vi "D-Lockin_JKISM.vi"(8 "error in (no error)":errorcluster, 11 "SweepControl":refnum<class "SweepControl.lvclass">) -> (0 "error out":errorcluster)   [LabVIEW 2016, in "Transport.lvclass"]
uses:
  Transport.lvclass
  <userlib>/LevyLab/LV to ITX/LVtoITX.lvclass
  SweepControl/SweepControl.lvclass
  Control Experiment/Control Experiment.lvclass
  <userlib>/LevyLab/Levylab Instruments/Instrument Types/Cryostat/Instrument.Cryostat.lvclass
panel:
  in  "OK":bool
  in  "Tab Control":enum32{"lockin/SG Control", "Data", "Other"}(tab)
  out "elapsed time (s) 2":u32=76
  out "T (mK) 2":dbl
  out "ramp rate 2":dbl=0.2 format="%#_13g"
  out "Field (T) 2":dbl=0.5 format="%#_13g"
  out "time b/w points (ms) 2":u32=76
  in  "Remote Lockin Address":string
  out "G4T":cluster{dbl[], dbl[]}[](graph)
  out "X Lockins":cluster{dbl[], dbl[]}[](graph)
  out "Y Lockins":cluster{dbl[], dbl[]}[](graph)
  # "This VI:\n1. does some initialization (e.g. file setup) (if outside i=0)\n2. add data to array and graph (for any i)\n3. write file when Stop = T"
  # "dynamically name the traces"
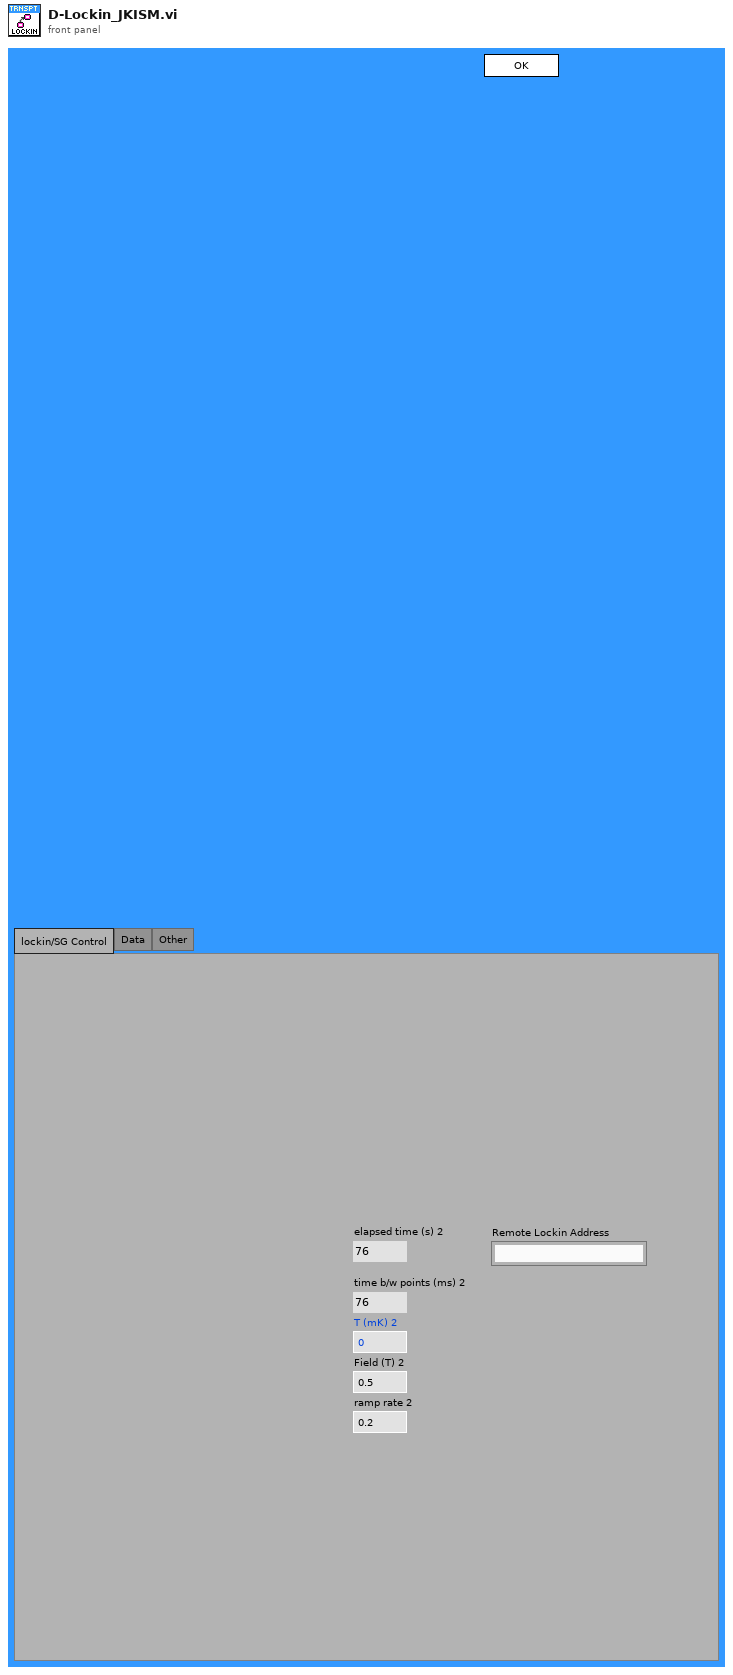
[diagram p1: front panel]
types:
  T1 = enum32{"Bad", "Idle", "Run top level", "Running"}
  T2 = enum32{"invalid app kind", "Development System", "Run Time System", "Student Edition", "Embedded LabVIEW", "Evaluation", "Custom"}
  T3 = enum32{"Invalid", "Standard", "Closed", "Hidden", "Minimized", "Maximized"}
  T4 = cluster{"Core":cluster{"Current VI Reference":refnum<vi>, "Close Panel on Exit?":bool}, "top level?":bool, "SweepControl":refnum<class "SweepControl.lvclass">, "Instrument":cluster{"Temperature":refnum<class "Instrument.Cryostat.lvclass">, "Magnet":refnum<class "Instrument.Cryostat.lvclass">, "Rotator":refnum<class "Instrument.Cryostat.lvclass">, "Level":refnum<class "Instrument.Cryostat.lvclass">}, "file":cluster{"path":path, "Experiment Folder":string, "device":string, "Comments":string}, "data":cluster{"Result X":dbl[], "Result Y":dbl[], "Data":cluster{"Y  Array":dbl[]}[], "wavenames":string[], "All Result X":dbl[][], "All Result Y":dbl[][]}, "lockin address":string, "Temperature (K)":dbl, "Field (T)":dbl, "ramp rate (T/min)":dbl, "Current Parameter":dbl}
  T5 = cluster{"Temperature":refnum<class "Instrument.Cryostat.lvclass">, "Magnet":refnum<class "Instrument.Cryostat.lvclass">, "Rotator":refnum<class "Instrument.Cryostat.lvclass">, "Level":refnum<class "Instrument.Cryostat.lvclass">}
  T6 = cluster{"Result X":dbl[], "Result Y":dbl[], "Data":cluster{"Y  Array":dbl[]}[], "wavenames":string[], "All Result X":dbl[][], "All Result Y":dbl[][]}
  T7 = cluster{"path":path, "Experiment Folder":string, "device":string, "Comments":string}
  T8 = cluster{"Current VI Reference":refnum<vi>, "Close Panel on Exit?":bool}
  T9 = typedef "AO-cluster.ctl" = cluster{"AO amp (V)":T10, "AO DC (V)":T11, "AO f (Hz)":T12, "AO phi (°)":T13, "function":T14, "I+":bool[]}
  T10 = typedef "AO_Amp-array.ctl" = dbl[]
  T11 = typedef "AO_DC-array.ctl" = dbl[]
  T12 = typedef "AO_f-array.ctl" = dbl[]
  T13 = typedef "AO_phi-array.ctl" = dbl[]
  T14 = typedef "Function-array.ctl" = T15[]
  T15 = typedef "Function-enum.ctl" = enum16{"Sine", "Triangle", "Square", "Sawtooth"}
  T16 = typedef "SweepControl.lvclass/ScanParamters.ctl" = T17[]
  T17 = typedef "SweepControl.lvclass/Cluster - ScanParamters.ctl" = cluster{"Start":dbl, "End":dbl, "Step":dbl, "Rate":dbl, "wait (ms)":u32, "Address":string, "channel":i32}
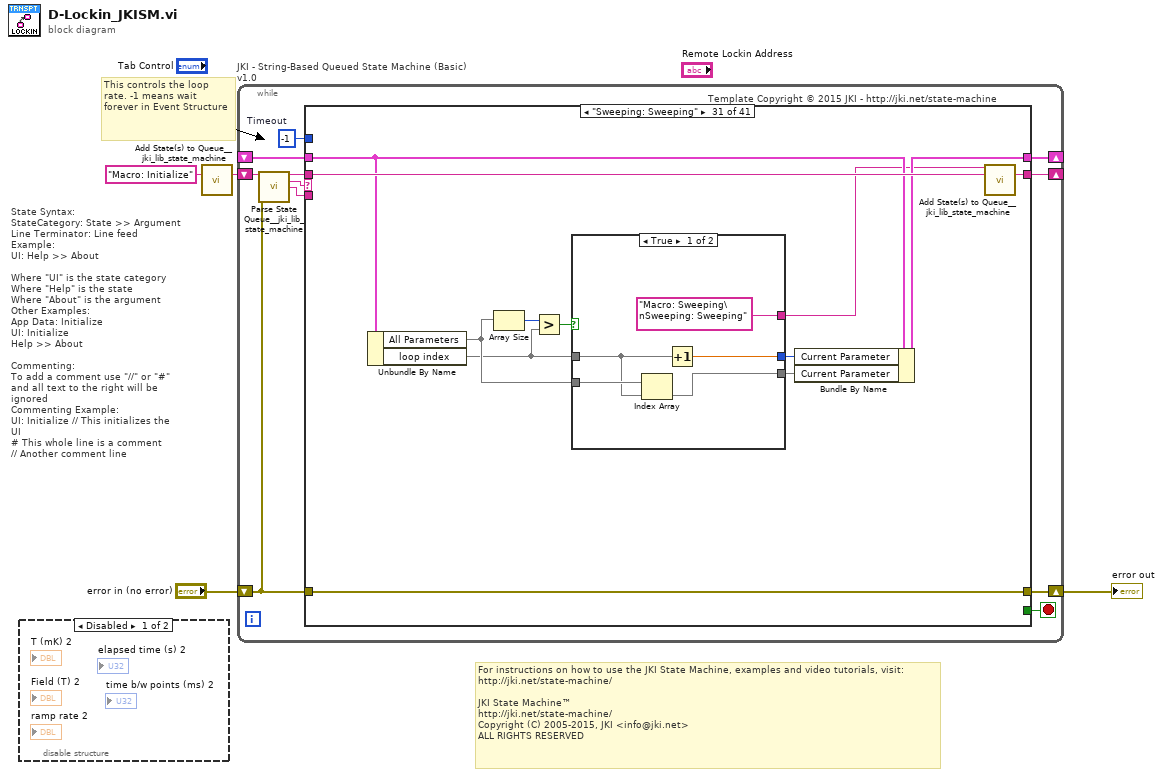
[diagram p0: block diagram]
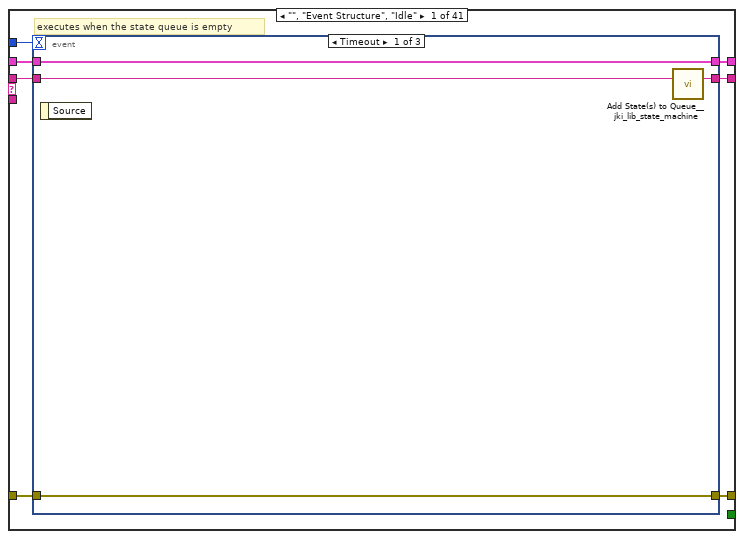
[diagram p3: hidden frame]
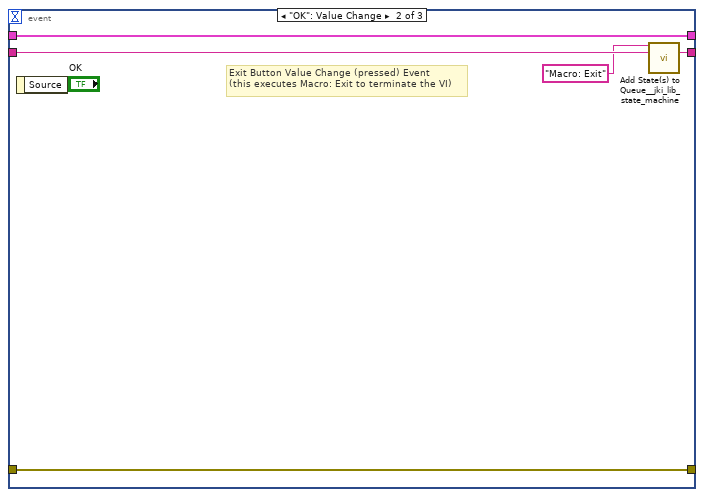
[diagram p4: hidden frame]
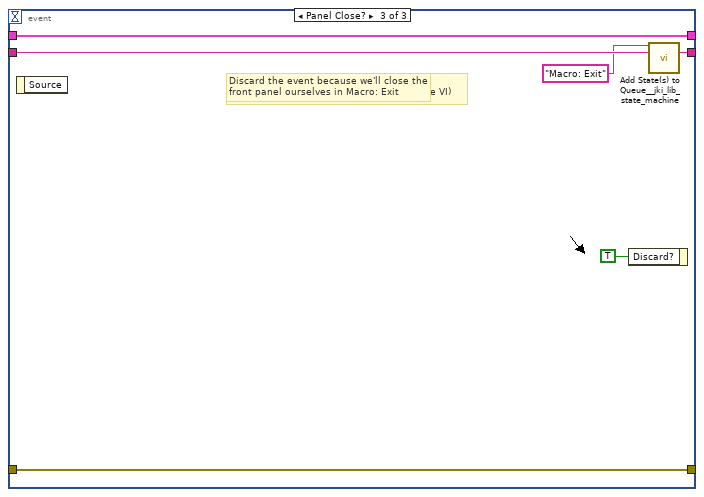
[diagram p5: hidden frame]
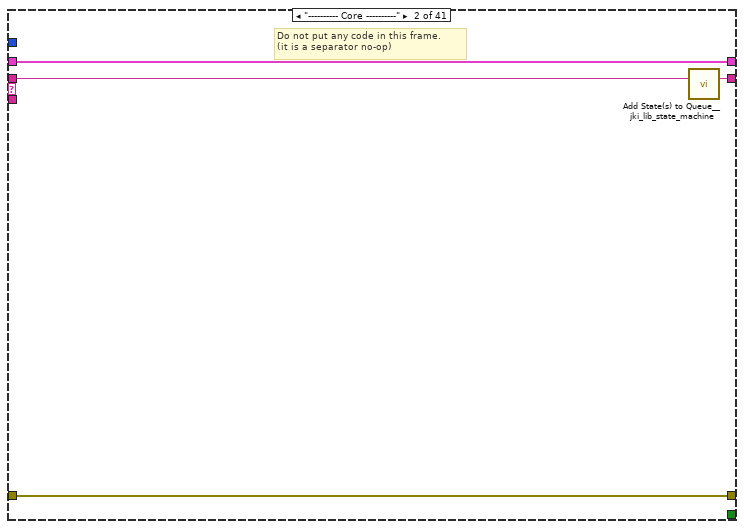
[diagram p6: hidden frame]
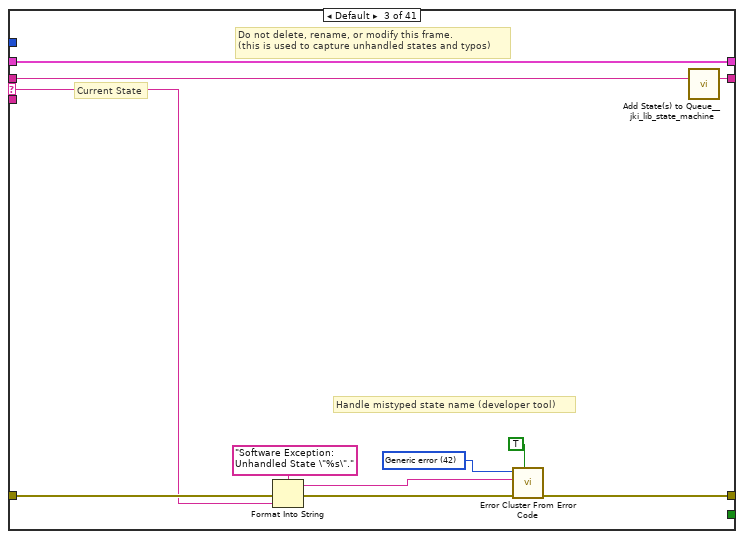
[diagram p7: hidden frame]
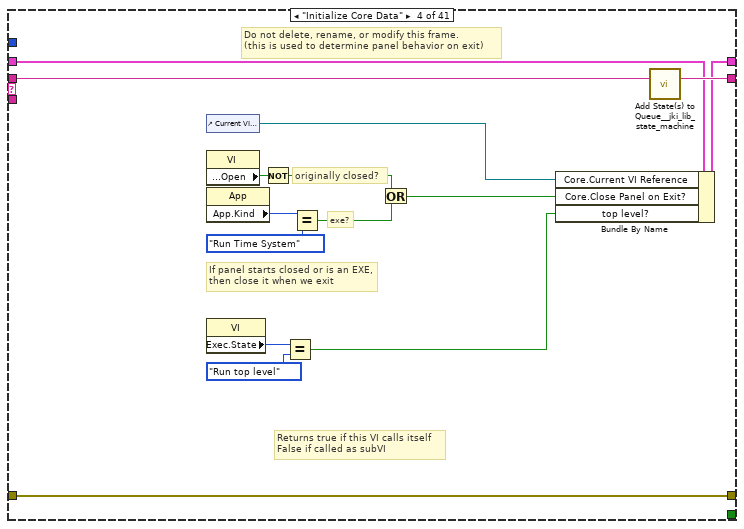
[diagram p8: hidden frame]
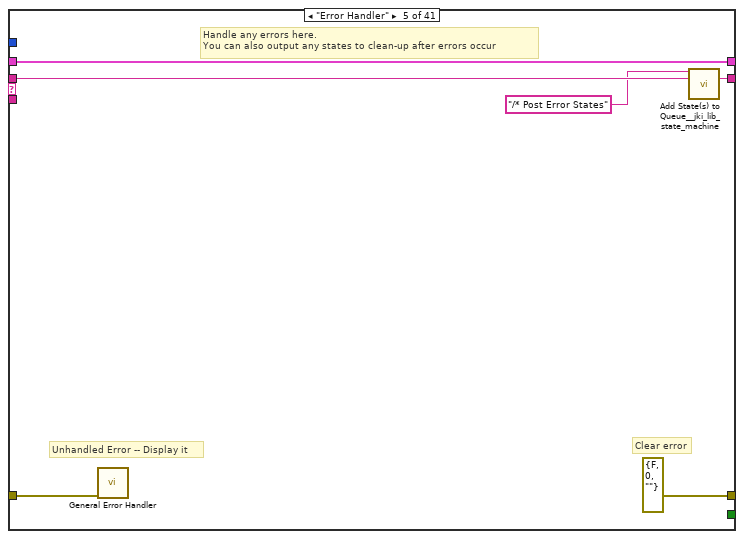
[diagram p9: hidden frame]
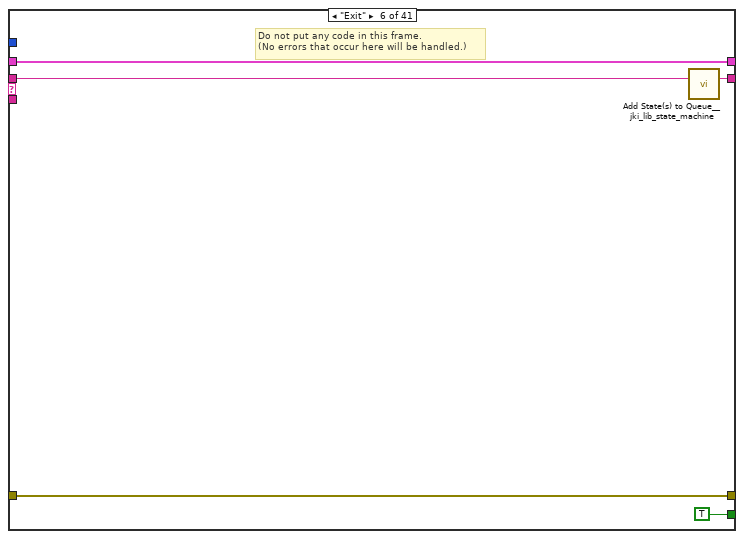
[diagram p10: hidden frame]
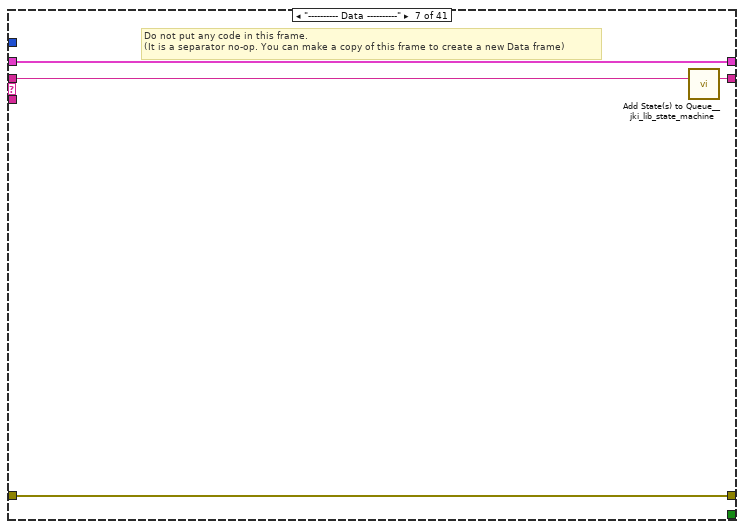
[diagram p11: hidden frame]
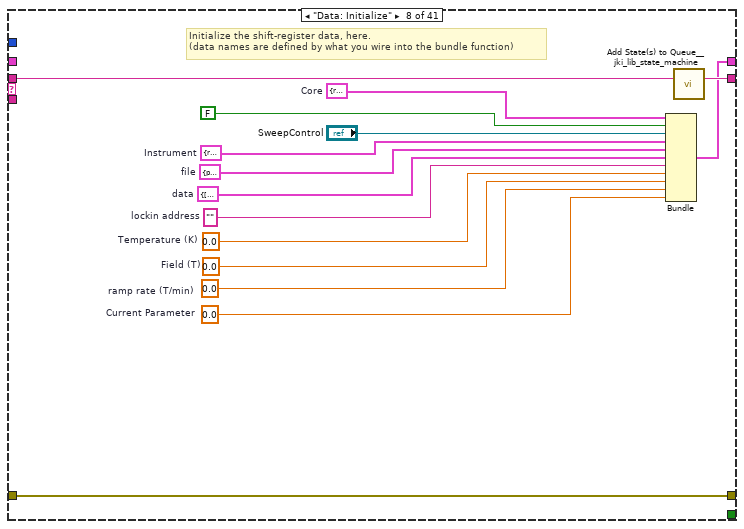
[diagram p12: hidden frame]
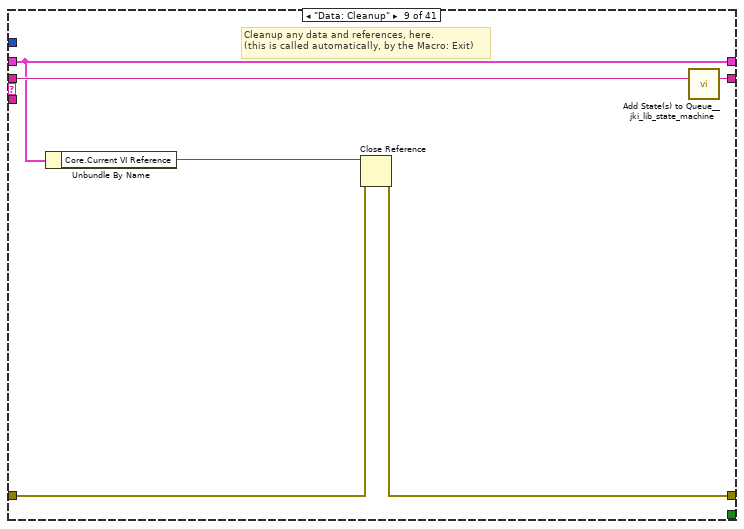
[diagram p13: hidden frame]
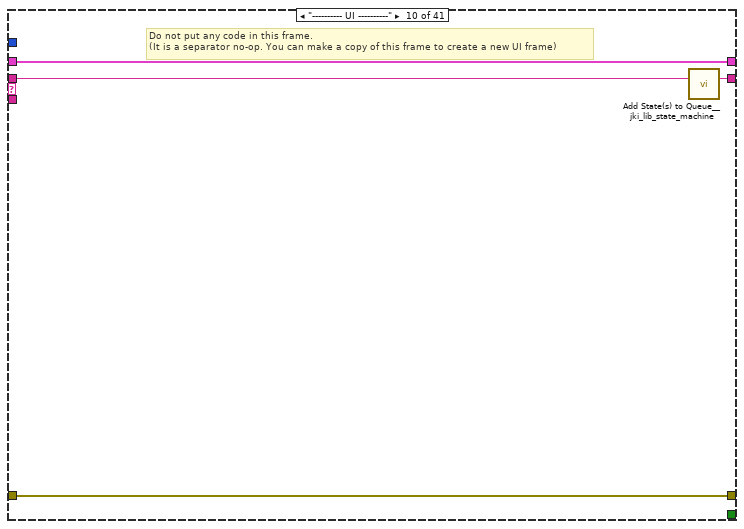
[diagram p14: hidden frame]
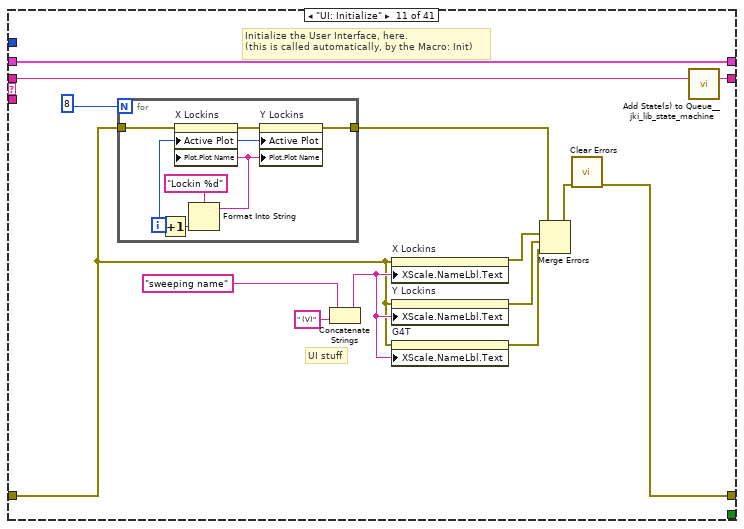
[diagram p15: hidden frame]
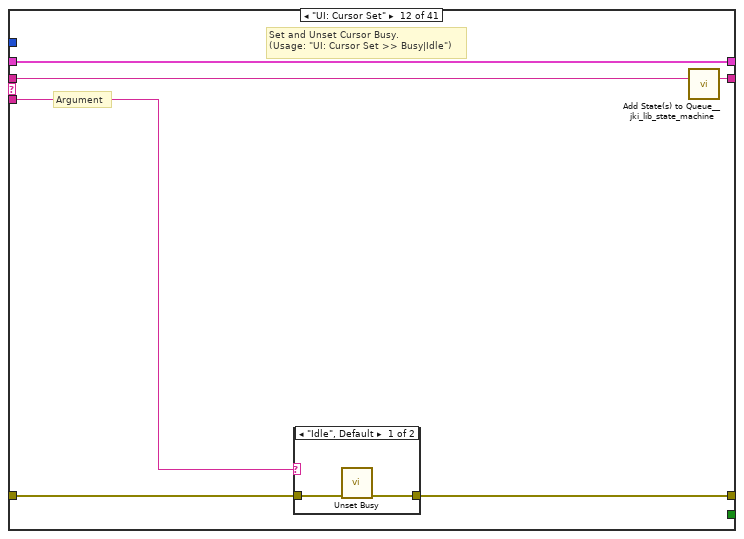
[diagram p16: hidden frame]
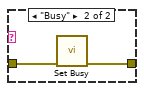
[diagram p17: hidden frame]
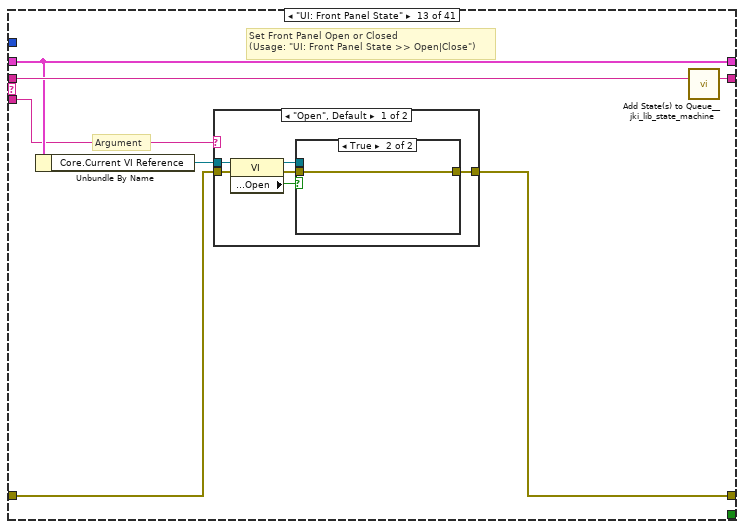
[diagram p18: hidden frame]
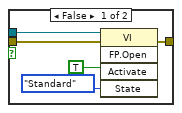
[diagram p19: hidden frame]
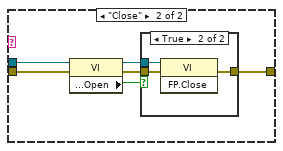
[diagram p20: hidden frame]
diagram:
  # "For instructions on how to use the JKI State Machine, examples and video tutorials, visit:\nhttp://jki.net/state-machine/\n\nJKI State Machine™\nhttp://jki.net/state-machine/\nCopyright (C) 2005-2015, JKI <info@jki.net>\nALL RIGHTS RESERVED"
  # "State Syntax:\nStateCategory: State >> Argument\nLine Terminator: Line feed\nExample:\nUI: Help >> About\n\nWhere \"UI\" is the state category\nWhere \"Help\" is the state\nWhere \"About\" is the argument\nOther Examples:\nApp Data: Initialize\nUI: Initialize\nHelp >> About\n\nCommenting:\nTo add a comment use \"//\" or \"#\" and all text to the right will be ignored\nCommenting Example:\nUI: Initialize // This initializes the UI\n# This whole line is a comment\n// Another comment line"
  # "This controls the loop rate. -1 means wait forever in Event Structure"
  n1 = disable-structure shown="Disabled" {
    frame Disabled {
    }
    frame Enabled {
    }
  }
  n2 = call <vilib>:"Add State(s) to Queue__jki_lib_state_machine.vi"("State(s) in (\"\")"="Macro: Initialize") -> ("States Out"=w4:string)  [unwired: 14 in]
  n3 = while "JKI - String-Based Queued State Machine (Basic) v1.0" {
    shift-right: [w8] -> _
    shift-left: _ -> [w7]
    shift-right: [w11] -> w1
    shift-left: "error in (no error)" -> [w5]
    shift-right: [w10] -> _
    shift-left: w4 -> [w12]
    stop <- w9 stop-if-true
    w6 = -1  # Timeout
    # "Template Copyright © 2015 JKI - http://jki.net/state-machine"
    n4 = call <vilib>:"Parse State Queue__jki_lib_state_machine.vi"("State Queue"=w12, "Error In (no error)"=w5) -> ("Remaining States"=w14:string, "Current State"=w15:string, "Arguments"=w13:string)  [unwired: 11 in]
    n5 = case shown="\"Sweeping: Sweeping\"" w15 {
      selector: w15 -> [_ _ w42 _ _ _ _ _ _ _ _ _ _ _ _ _ _ _ _ _ _ _ _ _ _ _ _ _ _ _ _ _ _ _ _ _ _ _ _ _ _]
      tunnel: w14 -> [w22 w41 w46 w67 w73 w78 w82 w97 w103 w107 w121 w134 w145 w171 w176 w181 w186 w191 w201 w205 w209 w213 w217 w225 w234 w238 w245 w275 w316 w320 w332 w356 w376 w382 w398 w414 w418 w435 w451 w464 w496]
      tunnel: w13 -> [_ _ _ _ _ _ _ _ _ _ _ w129 w139 _ _ _ _ _ _ _ _ _ _ _ _ _ _ _ _ _ _ _ _ _ _ _ _ _ _ _ _]
      tunnel: w7 -> [w20 w38 w44 w58 w70 w76 w79 _ w98 w104 w119 w132 w141 w168 w173 w178 w183 w188 w198 w202 w206 w210 w214 w223 w232 w235 w241 w269 w308 w317 w327 w354 w374 w377 w391 w406 w415 w432 w444 w453 w493]
      tunnel: [w19 w39 w48 w64 errorcluster {"status"=FALSE, "code"=0, "source"=""} ("error out") w75 w80 w94 w99 w105 w111 w130 w142 w169 w174 w179 w184 w189 w199 w203 w207 w211 w215 w218 w226 w236 w243 w271 w314 w318 w330 w348 w367 w379 w384 w412 w416 w433 w449 w462 w494] -> w11
      tunnel: w5 -> [w18 w39 w47 w64 w69 w75 w80 w94 w100 w105 w109 w131 w143 w169 w174 w179 w184 w189 w199 w203 w207 w211 w215 w219 w227 w236 w242 w272 w314 w318 w330 w350 w368 w380 w385 w412 w416 w433 w449 w462 w494]
      tunnel: [w21 w40 w45 w66 w72 w77 w81 w96 w102 w106 w120 w133 w144 w170 w175 w180 w185 w190 w200 w204 w208 w212 w216 w224 w233 w237 w244 w274 w315 w319 w331 w355 w375 w381 w397 w413 w417 w434 w450 w463 w495] -> w10
      tunnel: [_ _ _ _ _ TRUE _ _ _ _ _ _ _ _ _ _ _ _ _ _ _ _ _ _ _ _ _ _ _ _ _ _ _ _ _ _ _ _ _ _ _] -> w9
      tunnel: [w17 w38 w44 w65 w70 w76 w79 w95 w98 w104 w119 w132 w141 w168 w173 w178 w183 w188 w198 w202 w206 w210 w214 w222 w231 w235 w240 w273 w307 w317 w329 w354 w374 w377 w390 w406 w415 w431 w445 w452 w493] -> w8
      tunnel: w6 -> [w16 _ _ _ _ _ _ _ _ _ _ _ _ _ _ _ _ _ _ _ _ _ _ _ _ _ _ _ _ _ _ _ _ _ _ _ _ _ _ _ _]
      frame "", "Event Structure", "Idle" {
        # "executes when the state queue is empty"
        n6 = event shown="[0] Timeout" {
          selector: _ -> [_ _ _]
          dyn-events: _ -> [_ _ _]
          timeout: w16 -> [_ _ _]
          tunnel: w22 -> [w26 w31 w37]
          tunnel: [w25 w30 w36] -> w21
          tunnel: w20 -> [w23 w28 w34]
          tunnel: [w24 w29 w35] -> w19
          tunnel: w18 -> [w24 w29 w35]
          tunnel: [w23 w28 w34] -> w17
          event Timeout {
            n7 = event-data() -> ()  [unwired: 1 in, 1 out]
            n8 = call <vilib>:"Add State(s) to Queue__jki_lib_state_machine.vi"("State(s) in (\"\")"=w26) -> ("States Out"=w25:string)  [unwired: 14 in]
          }
          event "OK": Value Change {
            # "Exit Button Value Change (pressed) Event\n(this executes Macro: Exit to terminate the VI)"
            n9 = event-data() -> ()  [unwired: 1 in, 1 out]
            n10 = call <vilib>:"Add State(s) to Queue__jki_lib_state_machine.vi"("State(s) in Front (\"\")"="Macro: Exit", "State(s) in (\"\")"=w31) -> ("States Out"=w30:string)  [unwired: 13 in]
          }
          event Panel Close? {
            # "Discard the event because we'll close the front panel ourselves in Macro: Exit"
            # "Close Panel button (pressed) Event\n(this executes Macro: Exit to terminate the VI)"
            n11 = event-data() -> ()  [unwired: 1 in, 1 out]
            n12 = event-data("Discard?"=TRUE) -> ()  [unwired: 1 in, 1 out]
            n13 = call <vilib>:"Add State(s) to Queue__jki_lib_state_machine.vi"("State(s) in Front (\"\")"="Macro: Exit", "State(s) in (\"\")"=w37) -> ("States Out"=w36:string)  [unwired: 13 in]
          }
        }
      }
      frame "---------- Core ----------" {
        # "Do not put any code in this frame.\n(it is a separator no-op)"
        n14 = call <vilib>:"Add State(s) to Queue__jki_lib_state_machine.vi"("State(s) in (\"\")"=w41) -> ("States Out"=w40:string)  [unwired: 14 in]
      }
      frame Default {
        w51 = 42 items=["No error", "Argument error", "Memory is full", "Out of zone", "End of file", "File already open", "Generic file I/O error", "File not found", "File permission error", "Disk is full", "Duplicate path", "Too many files open", "System feature not enabled", "Resource file not found", "Cannot add resource", "Resource not found", "Image not found", "Image memory error", "Pen does not exist", "Config type invalid", "Config token not found", "Config parse error", "Config memory error", "Bad external code format", "Bad external code offset", "External code not present", "Null window", "Destroy window error", "Null menu", "Print aborted", "Bad print record", "Print driver error", "Windows error during printing", "Memory error during printing", "Print dialog error", "Generic print error", "Invalid device refnum", "Device not found", "Device parameter error", "Device unit error", "Cannot open device", "Device call aborted", "Generic error", "Cancelled by user", "Object ID too low", "Object ID too high", "Object not in heap", "Unknown heap", "Unknown object (invalid DefProc)", "Unknown object (DefProc not in table)", "Message out of range", "Invalid (null) method", "Unknown message", "Manager call not supported", "Bad address", "Network operation in progress", "Network operation timed out", "Connection is busy", "Network attribute not supported", "Network error", "Address in use", "System out of memory", "Connection aborted", "Connection refused", "Not connected", "Already connected", "Connection closed", "Initialization error (interapplication manager)", "Bad occurrence", "Wait on unbound occurrence handler", "Occurrence queue overflow", "Datalog type conflict", "Unused", "Unrecognized type (interapplication manager)", "Memory corrupt", "Failed to make temporary DLL", "Old CIN version", "Drag socket not found", "Failed to load drop-object", "Failed to register OLE object", "Failed to release OLE object", "Format specifier type mismatch", "Unknown format specifier", "Too few format specifiers", "Too many format specifiers", "Scan failed", "Newer CIN version", "Error converting to variant", "Runtime menu error", "Password tampered", "Variant attribute not found", "Incompatible variant data type", "Event data is not available", "Event Store is not present", "Occurrence is not found", "Event Queue is not created", "Event info is not available", "Refnum passed is NULL", "Error retrieving Class GUID", "Error retrieving CoClass GUID", "Error retrieving TypeLib GUID.", "Bad built application magic bytes.", "Specific driver is different from the specific driver associated with the Logical Name.", "There is no session opened to the class driver.", "Max Error", "MAX - Error with config objects", "MAX - Error loading configuration", "MAX - Group not supported"]
        # "Current State"
        # "Do not delete, rename, or modify this frame.\n(this is used to capture unhandled states and typos)"
        # "Handle mistyped state name (developer tool)"
        n15 = Format Into String(format string="Software Exception: Unhandled State \"%s\"." ("message"), error in=w47, w42) -> (resulting string=w50:string, error out=w49:errorcluster)  [unwired: 1 in]
        n16 = call <vilib>:"Error Cluster From Error Code.vi"("show call chain? (False)"=TRUE, "error in (no error)"=w49, "error message (\"\")"=w50, "error code (0)"=w51) -> ("error out"=w48:errorcluster)  [unwired: 5 in]
        n17 = call <vilib>:"Add State(s) to Queue__jki_lib_state_machine.vi"("State(s) in (\"\")"=w46) -> ("States Out"=w45:string)  [unwired: 14 in]
      }
      frame "Initialize Core Data" {
        # "Returns true if this VI calls itself\nFalse if called as subVI"
        # "Do not delete, rename, or modify this frame.\n(this is used to determine panel behavior on exit)"
        # "originally closed?"
        # "exe?"
        # "If panel starts closed or is an EXE, then close it when we exit"
        n18 = control-ref of="Current VI Reference"() -> (w56:refnum<vi>)
        n19 = property class="VI"() -> ("Front Panel.Open"=w63:bool)  [unwired: 2 in, 2 out]
        n20 = property class="App"() -> ("App.Kind"=w62:T2)  [unwired: 2 in, 2 out]
        n21 = property class="VI"() -> ("Exec.State"=w54:T1)  [unwired: 2 in, 2 out]
        n22 = Not(x=w63) -> (.not. x?=w60:bool)
        n23 = Equal?(x=w54, y=T1."Run top level" ("Execution:State")) -> (x = y?=w53:bool)
        n24 = Equal?(x=w62, y=T2."Run Time System" ("Application:Kind")) -> (x = y?=w59:bool)
        n25 = Or(x=w60, y=w59) -> (x .or. y?=w57:bool)
        n26 = Bundle By Name(cluster=w58, "Core.Current VI Reference"=w56, "Core.Close Panel on Exit?"=w57, "top level?"=w53) -> (w65:T4)
        n27 = call <vilib>:"Add State(s) to Queue__jki_lib_state_machine.vi"("State(s) in (\"\")"=w67) -> ("States Out"=w66:string)  [unwired: 14 in]
      }
      frame "Error Handler" {
        # "Unhandled Error -- Display it"
        # "Handle any errors here.\nYou can also output any states to clean-up after errors occur"
        # "Clear error"
        n28 = call <vilib>:"General Error Handler.vi"("error in (no error)"=w69) -> ()  [unwired: 10 in, 5 out]
        n29 = call <vilib>:"Add State(s) to Queue__jki_lib_state_machine.vi"("State(s) in Front (\"\")"="/* Post Error States", "State(s) in (\"\")"=w73) -> ("States Out"=w72:string)  [unwired: 13 in]
      }
      frame "Exit" {
        # "Do not put any code in this frame.\n(No errors that occur here will be handled.)"
        n30 = call <vilib>:"Add State(s) to Queue__jki_lib_state_machine.vi"("State(s) in (\"\")"=w78) -> ("States Out"=w77:string)  [unwired: 14 in]
      }
      frame "---------- Data ----------" {
        # "Do not put any code in this frame.\n(It is a separator no-op. You can make a copy of this frame to create a new Data frame)"
        n31 = call <vilib>:"Add State(s) to Queue__jki_lib_state_machine.vi"("State(s) in (\"\")"=w82) -> ("States Out"=w81:string)  [unwired: 14 in]
      }
      frame "Data: Initialize" {
        w85 = T5 {"Temperature"=refnum, "Magnet"=refnum, "Rotator"=refnum, "Level"=refnum}  # Instrument
        w87 = T6 {"Result X"=[], "Result Y"=[], "Data"=[], "wavenames"=[], "All Result X"=[], "All Result Y"=[]}  # data
        w84 = T7 {"path"=path "", "Experiment Folder"="", "device"="", "Comments"=""}  # file
        w89 = ""  # lockin address
        w90 = 0.0  # Current Parameter
        w83 = 0.0  # ramp rate (T/min)
        w91 = 0.0  # Field (T)
        w92 = 0.0  # Temperature (K)
        w93 = T8 {"Current VI Reference"=refnum, "Close Panel on Exit?"=FALSE}  # Core
        # "Initialize the shift-register data, here.\n(data names are defined by what you wire into the bundle function)"
        n32 = Bundle("Core"=w93, "top level?"=FALSE, "SweepControl"="SweepControl", "Instrument"=w85, "file"=w84, "data"=w87, "lockin address"=w89, "Temperature (K)"=w92, "Field (T)"=w91, "ramp rate (T/min)"=w83, "Current Parameter"=w90) -> (w95:T4)  [unwired: 1 in]
        n33 = call <vilib>:"Add State(s) to Queue__jki_lib_state_machine.vi"("State(s) in (\"\")"=w97) -> ("States Out"=w96:string)  [unwired: 14 in]
      }
      frame "Data: Cleanup" {
        # "Cleanup any data and references, here.\n(this is called automatically, by the Macro: Exit)"
        n34 = Unbundle By Name(w98) -> ("Core.Current VI Reference"=w101:refnum<vi>)
        n35 = Close Reference(reference=w101, error in (no error)=w100) -> (error out=w99:errorcluster)
        n36 = call <vilib>:"Add State(s) to Queue__jki_lib_state_machine.vi"("State(s) in (\"\")"=w103) -> ("States Out"=w102:string)  [unwired: 14 in]
      }
      frame "---------- UI ----------" {
        # "Do not put any code in this frame.\n(It is a separator no-op. You can make a copy of this frame to create a new UI frame)"
        n37 = call <vilib>:"Add State(s) to Queue__jki_lib_state_machine.vi"("State(s) in (\"\")"=w107) -> ("States Out"=w106:string)  [unwired: 14 in]
      }
      frame "UI: Initialize" {
        # "UI stuff"
        # "Initialize the User Interface, here.\n(this is called automatically, by the Macro: Init)"
        n38 = for {
          N: 8 -> [_]
          tunnel: [w122] -> w116
          tunnel: w109 -> [w127]
          i -> [w125]
          n39 = Increment(x=w125) -> (x+1=w123:i32)
          n40 = Format Into String(format string="Lockin %d", w123) -> (resulting string=w126:string)  [unwired: 2 in, 1 out]
          n41 = property on="X Lockins" class="XYGraph (strict)"(error in=w127, "Active Plot"=w125, "Plot.Plot Name"=w126) -> (error out=w124:errorcluster)  [unwired: 1 in, 1 out]
          n42 = property on="Y Lockins" class="XYGraph (strict)"(error in=w124, "Active Plot"=w125, "Plot.Plot Name"=w126) -> (error out=w122:errorcluster)  [unwired: 1 in, 1 out]
        }
        n43 = Concatenate Strings("sweeping name" ("string"), " (V)" ("string")) -> (w117:string)
        n44 = property on="X Lockins" class="XYGraph (strict)"(error in=w109, "XScale.NameLbl.Text"=w117) -> (error out=w115:errorcluster)  [unwired: 1 in, 1 out]
        n45 = property on="Y Lockins" class="XYGraph (strict)"(error in=w109, "XScale.NameLbl.Text"=w117) -> (error out=w114:errorcluster)  [unwired: 1 in, 1 out]
        n46 = property on="G4T" class="XYGraph (strict)"(error in=w109, "XScale.NameLbl.Text"=w117) -> (error out=w113:errorcluster)  [unwired: 1 in, 1 out]
        n47 = Merge Errors(w116, w115, w114, w113) -> (w112:errorcluster)
        n48 = call <vilib>:"Clear Errors.vi"("error in (no error)"=w112) -> ("error out"=w111:errorcluster)  [unwired: 5 in, 1 out]
        n49 = call <vilib>:"Add State(s) to Queue__jki_lib_state_machine.vi"("State(s) in (\"\")"=w121) -> ("States Out"=w120:string)  [unwired: 14 in]
      }
      frame "UI: Cursor Set" {
        # "Argument"
        # "Set and Unset Cursor Busy.\n(Usage: \"UI: Cursor Set >> Busy|Idle\")"
        n50 = case shown="\"Idle\", Default" w129 {
          tunnel: w131 -> [w136 w138]
          tunnel: [w135 w137] -> w130
          frame "Idle", Default {
            n51 = call <vilib>:"Unset Busy.vi"("error in (no error)"=w136) -> ("error out"=w135:errorcluster)  [unwired: 10 in]
          }
          frame "Busy" {
            n52 = call <vilib>:"Set Busy.vi"("error in (no error)"=w138) -> ("error out"=w137:errorcluster)  [unwired: 9 in, 1 out]
          }
        }
        n53 = call <vilib>:"Add State(s) to Queue__jki_lib_state_machine.vi"("State(s) in (\"\")"=w134) -> ("States Out"=w133:string)  [unwired: 14 in]
      }
      frame "UI: Front Panel State" {
        # "Argument"
        # "Set Front Panel Open or Closed\n(Usage: \"UI: Front Panel State >> Open|Close\")"
        n54 = Unbundle By Name(w141) -> ("Core.Current VI Reference"=w140:refnum<vi>)
        n55 = case shown="\"Open\", Default" w139 {
          tunnel: w143 -> [w149 w162]
          tunnel: [w151 w163] -> w142
          tunnel: w140 -> [w150 w160]
          frame "Open", Default {
            n56 = property class="VI"(reference=w150, error in=w149) -> (reference out=w147:refnum<vi>, error out=w148:errorcluster, "Front Panel.Open"=w146:bool)
            n57 = case shown="True" w146 {
              tunnel: [w154 w157] -> w151
              tunnel: w148 -> [w153 w157]
              tunnel: w147 -> [w152 _]
              frame False {
                n58 = invoke class="VI" method="FP.Open"(reference=w152, error in=w153, "Activate"=TRUE, "State"=T3."Standard") -> (error out=w154:errorcluster)  [unwired: 1 in, 4 out]
              }
              frame True {
              }
            }
          }
          frame "Close" {
            n59 = property class="VI"(reference=w160, error in=w162) -> (reference out=w159:refnum<vi>, error out=w161:errorcluster, "Front Panel.Open"=w158:bool)
            n60 = case shown="True" w158 {
              tunnel: [w164 w167] -> w163
              tunnel: w161 -> [w164 w166]
              tunnel: w159 -> [_ w165]
              frame False {
              }
              frame True {
                n61 = invoke class="VI" method="FP.Close"(reference=w165, error in=w166) -> (error out=w167:errorcluster)  [unwired: 1 in, 2 out]
              }
            }
          }
        }
        n62 = call <vilib>:"Add State(s) to Queue__jki_lib_state_machine.vi"("State(s) in (\"\")"=w145) -> ("States Out"=w144:string)  [unwired: 14 in]
      }
      frame "---------- Macro ----------" {
        # "Do not put any code in this frame.\n(It is a separator no-op. You can make a copy of this frame to create a new Macro frame)"
        n63 = call <vilib>:"Add State(s) to Queue__jki_lib_state_machine.vi"("State(s) in (\"\")"=w171) -> ("States Out"=w170:string)  [unwired: 14 in]
      }
      frame "Macro: Initialize" {
        w172 = "Data: Initialize\nInitialize Core Data\nUI: Initialize\nUI: Front Panel State >> Open\nMacro: Sweep"  # Data: Initialize Initialize Core Data UI: Initialize UI: Front Panel State >> Open Macro: Sweep
        # "Initialization Macro\n(This is called once, when the VI starts)"
        n64 = call <vilib>:"Add State(s) to Queue__jki_lib_state_machine.vi"("State(s) in Front (\"\")"=w172, "State(s) in (\"\")"=w176) -> ("States Out"=w175:string)  [unwired: 13 in]
      }
      frame "Macro: Sweep" {
        n65 = call <vilib>:"Add State(s) to Queue__jki_lib_state_machine.vi"("State(s) in Front (\"\")"="Sweep: Get\nSweep: Get Remote\nSweep: Define Sweep\nSweeping: Sweeping", "State(s) in (\"\")"=w181) -> ("States Out"=w180:string)  [unwired: 13 in]
      }
      frame "Macro: Sweeping" {
        n66 = call <vilib>:"Add State(s) to Queue__jki_lib_state_machine.vi"("State(s) in Front (\"\")"="Sweeping: Set Parameter\nSweeping: Wait\nSweeping: Wait New AI\nSweeping: Get Result\nSweeping: Plot", "State(s) in (\"\")"=w186) -> ("States Out"=w185:string)  [unwired: 13 in]
      }
      frame "Macro: Save" {
        n67 = call <vilib>:"Add State(s) to Queue__jki_lib_state_machine.vi"("State(s) in Front (\"\")"="File: Prepare 0D Data\nFile: Prepare 1D Data\nFile: Prepare 2D Data\nFile: Save ITX", "State(s) in (\"\")"=w191) -> ("States Out"=w190:string)  [unwired: 13 in]
      }
      frame "Macro: Exit" {
        # "Exit Macro\n(This is called once, when the VI exits)"
        n68 = Unbundle By Name(w198) -> ("Core.Close Panel on Exit?"=w197:bool)
        n69 = Select(t="UI: Front Panel State >> Close", s=w197, f="") -> (s? t:f=w194:string)
        n70 = call <vilib>:"Add State(s) to Queue__jki_lib_state_machine.vi"("State(s) in (\"\")"=w194, "State(s) at Back (\"\")"="Data: Cleanup\nExit") -> ("States Out"=w192:string)  [unwired: 13 in]
        n71 = call <vilib>:"Add State(s) to Queue__jki_lib_state_machine.vi"("State(s) in Front (\"\")"=w192, "State(s) in (\"\")"=w201) -> ("States Out"=w200:string)  [unwired: 13 in]
      }
      frame "---------- Lockin ----------" {
        # "Template Separator\n(You can make a copy of, or modify, this frame)"
        n72 = call <vilib>:"Add State(s) to Queue__jki_lib_state_machine.vi"("State(s) in (\"\")"=w205) -> ("States Out"=w204:string)  [unwired: 14 in]
      }
      frame "Lockin: 1" {
        # "Your code here.\n(You can make a copy of, or modify, this frame)"
        n73 = call <vilib>:"Add State(s) to Queue__jki_lib_state_machine.vi"("State(s) in (\"\")"=w209) -> ("States Out"=w208:string)  [unwired: 14 in]
      }
      frame "Lockin: 2" {
        # "Your code here.\n(You can make a copy of, or modify, this frame)"
        n74 = call <vilib>:"Add State(s) to Queue__jki_lib_state_machine.vi"("State(s) in (\"\")"=w213) -> ("States Out"=w212:string)  [unwired: 14 in]
      }
      frame "---------- Instrument ----------" {
        # "Template Separator\n(You can make a copy of, or modify, this frame)"
        n75 = call <vilib>:"Add State(s) to Queue__jki_lib_state_machine.vi"("State(s) in (\"\")"=w217) -> ("States Out"=w216:string)  [unwired: 14 in]
      }
      frame "Instrument: Get Temperature" {
        n76 = Unbundle By Name(w223) -> ("Instrument.Temperature"=w221:refnum<class "Instrument.Cryostat.lvclass">)
        n77 = call-dynamic "Get Temperature.vi"("error in (no error)"=w219, "Instrument.Cryostat in"=w221) -> ("error out"=w218:errorcluster, "Temperature (K)"=w220:dbl)  [unwired: 6 in, 2 out]
        n78 = Bundle By Name(cluster=w223, "Temperature (K)"=w220) -> (w222:T4)
        n79 = call <vilib>:"Add State(s) to Queue__jki_lib_state_machine.vi"("State(s) in (\"\")"=w225) -> ("States Out"=w224:string)  [unwired: 14 in]
      }
      frame "Instrument: Get Magnet" {
        n80 = Unbundle By Name(w232) -> ("Instrument.Magnet"=w230:refnum<class "Instrument.Cryostat.lvclass">)
        n81 = call-dynamic "Get Magnet.vi"("error in (no error)"=w227, "Instrument.Cryostat in"=w230) -> ("error out"=w226:errorcluster, "B Field (T)"=w229:dbl)  [unwired: 6 in, 2 out]
        n82 = Bundle By Name(cluster=w232, "Field (T)"=w229, "ramp rate (T/min)"=0.0) -> (w231:T4)
        n83 = call <vilib>:"Add State(s) to Queue__jki_lib_state_machine.vi"("State(s) in (\"\")"=w234) -> ("States Out"=w233:string)  [unwired: 14 in]
      }
      frame "---------- Sweep ----------" {
        # "Template Separator\n(You can make a copy of, or modify, this frame)"
        n84 = call <vilib>:"Add State(s) to Queue__jki_lib_state_machine.vi"("State(s) in (\"\")"=w238) -> ("States Out"=w237:string)  [unwired: 14 in]
      }
      frame "Sweep: Get" {
        n85 = Unbundle By Name(w241) -> ("top level?"=w239:bool)
        n86 = case shown="False" w239 {
          tunnel: [w255 w264] -> w243
          tunnel: w242 -> [w249 w265]
          tunnel: w241 -> [w248 w268]
          tunnel: [w247 w267] -> w240
          frame False {
            # "#todo\nThese need to be read from the FGV when\nthis is called as top level VI (do not get from the class\nwire)"
            n87 = Unbundle By Name(w248) -> ("SweepControl"=w260:refnum<class "SweepControl.lvclass">)
            n88 = call-dynamic "Read path.vi"("error in (no error)"=w249, "SweepControl in"=w260) -> ("error out"=w258:errorcluster, "path"=w257:path, "SweepControl out"=w259:refnum<class "SweepControl.lvclass">)  [unwired: 7 in]
            n89 = call-dynamic "Read device.vi"("error in (no error)"=w258, "SweepControl in"=w259) -> ("error out"=w254:errorcluster, "device"=w256:string, "SweepControl out"=w253:refnum<class "SweepControl.lvclass">)  [unwired: 7 in]
            n90 = call-dynamic "Read Comments.vi"("error in (no error)"=w254, "SweepControl in"=w253) -> ("error out"=w251:errorcluster, "Comments"=w250:string, "SweepControl out"=w252:refnum<class "SweepControl.lvclass">)  [unwired: 7 in]
            n91 = call-dynamic "Read Instrument.vi"("error in (no error)"=w251, "SweepControl in"=w252) -> ("error out"=w255:errorcluster, "Instrument"=w246:T5)  [unwired: 7 in, 1 out]
            n92 = Bundle By Name(cluster=w248, "file.path"=w257, "file.device"=w256, "file.Comments"=w250, "Instrument"=w246) -> (w247:T4)
          }
          frame True {
            # "#todo\nThese need to be read from the FGV when\nthis is called as top level VI (do not get from the class\nwire)"
            # "TOP LEVEL VI"
            n93 = Unbundle By Name(w268) -> ("lockin address"=w266:string)
            n94 = call "Initialize Experiment.vi"("lockin address"=w266, "error in (no error)"=w265) -> ("error out"=w264:errorcluster, "Comments"=w261:string, "device"=w262:string, "path"=w263:path)  [unwired: 6 in]
            n95 = Bundle By Name(cluster=w268, "file.path"=w263, "file.device"=w262, "file.Comments"=w261) -> (w267:T4)
          }
        }
        n96 = call <vilib>:"Add State(s) to Queue__jki_lib_state_machine.vi"("State(s) in (\"\")"=w245) -> ("States Out"=w244:string)  [unwired: 14 in]
      }
      frame "Sweep: Get Remote" {
        # "#todo\nexperiment folder name should be generated automatically\n(### - Calling VI - Something Descriptive)"
        n97 = Unbundle By Name(w269) -> ("top level?"=w270:bool)
        n98 = case shown="False" w270 {
          tunnel: w269 -> [w292 w298]
          tunnel: [w291 w299] -> w273
          tunnel: w272 -> [w294 w297]
          tunnel: [w282 w297] -> w271
          frame False {
            n99 = Unbundle By Name(w292) -> ("SweepControl"=w290:refnum<class "SweepControl.lvclass">)
            n100 = call-dynamic "Read Channels_ AO.vi"("error in (no error)"=w294, "SweepControl in"=w290) -> ("error out"=w281:errorcluster, "Channels: AO"=w279:T9, "SweepControl out"=w280:refnum<class "SweepControl.lvclass">)  [unwired: 7 in]
            n101 = call-dynamic "Read Experiment folder name.vi"("error in (no error)"=w281, "SweepControl in"=w280) -> ("error out"=w287:errorcluster, "Experiment folder name"=w293:string, "SweepControl out"=w286:refnum<class "SweepControl.lvclass">)  [unwired: 7 in]
            n102 = call-dynamic "Read Sorted scan parameters.vi"("error in (no error)"=w287, "SweepControl in"=w286) -> ("error out"=w282:errorcluster, "Sorted scan parameters"=w289:cluster{T16}[])  [unwired: 7 in, 1 out]
            n103 = Index Array(array=w289) -> (element=w288:cluster{T16})  [unwired: 1 in]
            n104 = Unbundle(w288) -> (w278:T16)
            n105 = Index Array(array=w278) -> (element=w277:T17)  [unwired: 1 in]
            n106 = Unbundle By Name(w277) -> ("Start"=w285:dbl, "End"=w284:dbl, "Step"=w276:dbl, "channel"=w283:i32)
            n107 = Bundle By Name(cluster=w292, "Temperature (K)"=w279, "file.Experiment Folder"=w293, "Current Parameter"=w277) -> (w291:T4)
            n108 = local write item#-1(w284) -> ()
            n109 = local write item#-1(w283) -> ()
            n110 = local write item#-1(w276) -> ()
            n111 = local write item#-1(w285) -> ()
          }
          frame True {
            n112 = Bundle By Name(cluster=w298) -> (w299:T4, "file.Experiment Folder"=w296:string, "Current Parameter"=w302:dbl, "Current Parameter"=w301:dbl, "Step"=w300:dbl, "channel"=w295:i32)
          }
        }
        n113 = call <vilib>:"Add State(s) to Queue__jki_lib_state_machine.vi"("State(s) in (\"\")"=w275) -> ("States Out"=w274:string)  [unwired: 14 in]
      }
      frame "Sweep: Define Sweep" {
        n114 = Unbundle By Name(w308) -> ("End"=w311, "Start"=w310, "Step"=w309)
        n115 = call <userlib>:"Max_Min_conversion.vi"("Min"=w310, "Max"=w311) -> ("offset"=w313:dbl, "Amplitude"=w312:dbl)  [unwired: 8 in]
        n116 = call <userlib>:"Ramp.vi"("step size"=w309, "offset"=w313, "amplitude"=w312) -> ("Waveform Graph"=w306:dbl[], "phase"=w303:dbl, "function (ramp)"=w305:enum16{"Ramp", "Triangle", "Sine"}, "cycles (1,2,...)"=w304:i32)  [unwired: 3 in, 2 out]
        n117 = Bundle By Name(cluster=w308, "Current Parameter"=w306) -> (w307:T4)
        n118 = call <vilib>:"Add State(s) to Queue__jki_lib_state_machine.vi"("State(s) in (\"\")"=w316) -> ("States Out"=w315:string)  [unwired: 14 in]
      }
      frame "---------- Sweeping ----------" {
        # "Template Separator\n(You can make a copy of, or modify, this frame)"
        n119 = call <vilib>:"Add State(s) to Queue__jki_lib_state_machine.vi"("State(s) in (\"\")"=w320) -> ("States Out"=w319:string)  [unwired: 14 in]
      }
      frame "Sweeping: Sweeping" {
        n120 = Unbundle By Name(w327) -> ("All Parameters"=w324, "loop index"=w323)
        n121 = Array Size(array=w324) -> (size(s)=w326:i32)
        n122 = Greater?(x=w326, y=w323) -> (0:w322:bool)
        n123 = case shown="True" w322 {
          tunnel: [w337 -1] -> w328
          tunnel: [w336 w344] -> w325
          tunnel: w324 -> [w335 w345]
          tunnel: w323 -> [w334 _]
          tunnel: ["Macro: Sweeping\nSweeping: Sweeping" w338] -> w321
          frame True {
            n124 = Index Array(array=w335, index=w334) -> (element=w336)
            n125 = Increment(x=w334) -> (x+1=w337:dbl)
          }
          frame False {
            n126 = Index Array(array=w345) -> (element=w344)  [unwired: 1 in]
            n127 = Select(t="Sweeping: Set Parameter", f="") -> (s=w343:bool, s? t:f=w339:string)
            n128 = call <vilib>:"Add State(s) to Queue__jki_lib_state_machine.vi"("State(s) in Front (\"\")"=w339, "State(s) at Back (\"\")"="Macro: Save\nMacro: Exit") -> ("States Out"=w338:string)  [unwired: 13 in]
          }
        }
        n129 = Bundle By Name(cluster=w327, "Current Parameter"=w328, "Current Parameter"=w325) -> (w329:T4)
        n130 = call <vilib>:"Add State(s) to Queue__jki_lib_state_machine.vi"("State(s) in Front (\"\")"=w321, "State(s) in (\"\")"=w332) -> ("States Out"=w331:string)  [unwired: 13 in]
      }
      frame "Sweeping: Set Parameter" {
        # "#todo\nlockin address and \"physical channel\" should be stored in same way (as part of instrument\nconfiguration)"
        n131 = Unbundle By Name(w354) -> ("lockin address"=w347:string, "Channels: AO"=w353, "channel"=w352, "Current Parameter"=w351:dbl)
        n132 = case shown="\"Vsg\", Default" w349 {
          tunnel: w353 -> [w362 _]
          tunnel: w352 -> [w361 _]
          tunnel: w351 -> [w360 w365]
          tunnel: [w359 w363] -> w348
          tunnel: w350 -> [w358 w364]
          tunnel: w347 -> [w357 _]
          frame "Vsg", Default {
            n133 = call <userlib>:"configAO_DC.vi"("address"=w357, "error in (no error)"=w358, "new DC (V)"=w360, "AO Channel"=w361, "Channels: AO"=w362) -> ("error out"=w359:errorcluster)  [unwired: 5 in, 1 out]
          }
          frame "Vbg" {
            n134 = call <vilib>:"Voltage Update.vi"("error in (no error)"=w364, "Voltage Output"=w365) -> ("error out"=w363:errorcluster, "Physical Channel"=w366:tag)  [unwired: 7 in, 1 out]
          }
        }
        n135 = call <vilib>:"Add State(s) to Queue__jki_lib_state_machine.vi"("State(s) in (\"\")"=w356) -> ("States Out"=w355:string)  [unwired: 14 in]
      }
      frame "Sweeping: Wait" {
        n136 = Unbundle By Name(w374) -> ("loop index"=w370)
        n137 = Equal To 0?(x=w370) -> (x = 0?=w373:bool)
        n138 = Select(s=w373) -> (t=w371:dbl, f=w372:dbl, s? t:f=w369:dbl)
        n139 = call <userlib>:"Wait (ms)__ogtk.vi"("error in (no error)"=w368, "milliseconds to wait"=w369) -> ("error out"=w367:errorcluster)  [unwired: 8 in, 1 out]
        n140 = call <vilib>:"Add State(s) to Queue__jki_lib_state_machine.vi"("State(s) in (\"\")"=w376) -> ("States Out"=w375:string)  [unwired: 14 in]
      }
      frame "Sweeping: Wait New AI" {
        n141 = Unbundle By Name(w377) -> ("lockin address"=w378:string)
        n142 = call <userlib>:"waitForNewWaveforms.vi"("address"=w378, "error in (no error)"=w380) -> ("error out"=w379:errorcluster)  [unwired: 8 in, 1 out]
        n143 = call <vilib>:"Add State(s) to Queue__jki_lib_state_machine.vi"("State(s) in (\"\")"=w382) -> ("States Out"=w381:string)  [unwired: 14 in]
      }
      frame "Sweeping: Get Result" {
        n144 = Unbundle By Name(w391) -> ("data.All Result X"=w393:dbl[][], "data.All Result Y"=w392:dbl[][], "lockin address"=w396:string)
        n145 = call <userlib>:"readResults.vi"("address"=w396, "error in (no error)"=w385) -> ("error out"=w384:errorcluster, "Results"=w383:dbl[][])  [unwired: 7 in, 1 out]
        n146 = Array Size(array=w383) -> (size(s)=w395:i32[])
        n147 = Index Array(array=w395) -> (element=w394:i32)  [unwired: 1 in]
        n148 = for {
          N: w394 -> [_]
          tunnel: w383 -> [w404]
          tunnel: [w402] -> w389 mode=indexing
          tunnel: [w401] -> w388 mode=indexing
          i -> [w403]
          w399 = 1  # y
          w400 = 0  # x
          # "extract x and y"
          n149 = Index Array(array=w404, index (row) #1=w403, index (col) #1=w400, index (row) #2=w403, index (col) #2=w399) -> (element #1=w402:dbl, element #2=w401:dbl)
        }
        n150 = Build Array (concatenate)(w393, w389) -> (w386:dbl[][])
        n151 = Build Array (concatenate)(w392, w388) -> (w387:dbl[][])
        n152 = Bundle By Name(cluster=w391, "data.All Result X"=w386, "data.Result X"=w389, "data.All Result Y"=w387, "data.Result Y"=w388) -> (w390:T4)
        n153 = call <vilib>:"Add State(s) to Queue__jki_lib_state_machine.vi"("State(s) in (\"\")"=w398) -> ("States Out"=w397:string)  [unwired: 14 in]
      }
      frame "Sweeping: Plot" {
        # "#todo:\nget I, V1, V2 from Control Experiment"
        n154 = Unbundle By Name(w406) -> ("loop index"=w409, "data.Result X"=w407:dbl[], "Current Parameter"=w405:dbl)
        n155 = Equal To 0?(x=w409) -> (x = 0?=w408:bool)
        n156 = call "GraphLockin_vs_Parameter.vi"("reset?"=w408, "Parameter"=w405, "X[ ]"=w407) -> ("Y vs Parameter"=→"X Lockins" →"Y Lockins":cluster{dbl[], dbl[]}[], "X vs Parameter"=→"G4T":cluster{dbl[], dbl[]}[])  [unwired: 5 in, 2 out]
        n157 = call <vilib>:"Add State(s) to Queue__jki_lib_state_machine.vi"("State(s) in (\"\")"=w414) -> ("States Out"=w413:string)  [unwired: 14 in]
      }
      frame "---------- File ----------" {
        # "Template Separator\n(You can make a copy of, or modify, this frame)"
        n158 = call <vilib>:"Add State(s) to Queue__jki_lib_state_machine.vi"("State(s) in (\"\")"=w418) -> ("States Out"=w417:string)  [unwired: 14 in]
      }
      frame "File: Prepare 0D Data" {
        # "#todo\nthese should be made dynamically from \"get/set parameter\""
        n159 = Unbundle By Name(w432) -> ("data.Data"=w430:cluster{"Y  Array":dbl[]}[], "data.wavenames"=w429:string[], "Temperature (K)"=w423:dbl, "Field (T)"=w422:dbl, "ramp rate (T/min)"=w421:dbl)
        n160 = Get Date/Time In Seconds() -> (seconds since 1Jan1904=w425:timestamp)
        n161 = To Double Precision Float(number=w425) -> (double precision float=w424:dbl)
        n162 = Build Array(w424, w423, w422, w421) -> (w419:dbl[])
        n163 = for {
          tunnel: [w437] -> w420 mode=concatenating
          tunnel: w419 -> [w436] mode=indexing
          # "build cluster array"
          n164 = Build Array(w436) -> (w438:dbl[])
          n165 = Build Cluster Array(w438) -> (w437:cluster{dbl[]}[])
        }
        n166 = Build Array (concatenate)(w430, w420) -> (w427:cluster{"Y  Array":dbl[]}[])
        n167 = Build Array (concatenate)(w429, string[] ["time", "T", "B", "B_rate"] ("wavenames (.Vx, etc)")) -> (w428:string[])
        n168 = Bundle By Name(cluster=w432, "data.Data"=w427, "data.wavenames"=w428) -> (w431:T4)
        n169 = call <vilib>:"Add State(s) to Queue__jki_lib_state_machine.vi"("State(s) in (\"\")"=w435) -> ("States Out"=w434:string)  [unwired: 14 in]
      }
      frame "File: Prepare 1D Data" {
        # "#todo\nthese should be made dynamically from \"get/set parameter\"\n(?)"
        # "Template Separator\n(You can make a copy of, or modify, this frame)"
        n170 = Unbundle By Name(w444) -> ("data.Data"=w448:cluster{"Y  Array":dbl[]}[], "data.wavenames"=w447:string[], "All Parameters"=w442)
        n171 = Build Cluster Array(w442) -> (w441:cluster{"All Parameters":void}[])
        n172 = Build Array() -> (w443:void[], w440:dbl)
        n173 = Build Array (concatenate)(w447, w443) -> (w439:string[])
        n174 = Build Array (concatenate)(w448, w441) -> (w446:cluster{"Y  Array":dbl[]}[])
        n175 = Bundle By Name(cluster=w444, "data.Data"=w446, "data.wavenames"=w439) -> (w445:T4)
        n176 = call <vilib>:"Add State(s) to Queue__jki_lib_state_machine.vi"("State(s) in (\"\")"=w451) -> ("States Out"=w450:string)  [unwired: 14 in]
      }
      frame "File: Prepare 2D Data" {
        # "dynamically format lockin data cluster & wavenames\n--> less wires & cleaner code\n--> number of channels is scalable"
        n177 = Unbundle By Name(w453) -> ("data.Data"=w461:cluster{"Y  Array":dbl[]}[], "data.wavenames"=w460:string[], "data.All Result X"=w457:dbl[][], "data.All Result Y"=w456:dbl[][])
        n178 = flat-sequence {
          tunnel: w457 -> [w474]
          tunnel: w456 -> [w473]
          tunnel: [w466] -> w454
          tunnel: [w465] -> w455
          frame #0 {
            # "build cluster array(s) of multiple 1D data, dynamically name waves"
            n179 = Transpose 2D Array(2D array=w474) -> (transposed array=w472:dbl[][])
            n180 = Transpose 2D Array(2D array=w473) -> (transposed array=w471:dbl[][])
            n181 = for {
              tunnel: w472 -> [w485] mode=indexing
              tunnel: w471 -> [w484] mode=indexing
              tunnel: [w483] -> w470 mode=concatenating
              tunnel: [w482] -> w469 mode=concatenating
              tunnel: [w477] -> w468 mode=indexing
              tunnel: [w476] -> w467 mode=indexing
              i -> [w479]
              n182 = Increment(x=w479) -> (x+1=w475:i32)
              n183 = Number To Decimal String(number=w475) -> (decimal integer string=w478:string)  [unwired: 1 in]
              n184 = Concatenate Strings("X" ("wavenames"), w478) -> (w477:string)
              n185 = Concatenate Strings("Y" ("wavenames"), w478) -> (w476:string)
              n186 = Build Cluster Array(w485) -> (w483:cluster{dbl[]}[])
              n187 = Build Cluster Array(w484) -> (w482:cluster{dbl[]}[])
            }
            n188 = Interleave 1D Arrays(w470, w469) -> (w465:cluster{dbl[]}[])
            n189 = Interleave 1D Arrays(w468, w467) -> (w466:string[])
          }
        }
        n190 = Build Array (concatenate)(w461, w455) -> (w458:cluster{"Y  Array":dbl[]}[])
        n191 = Build Array (concatenate)(w460, w454) -> (w459:string[])
        n192 = Bundle By Name(cluster=w453, "data.Data"=w458, "data.wavenames"=w459) -> (w452:T4)
        n193 = call <vilib>:"Add State(s) to Queue__jki_lib_state_machine.vi"("State(s) in (\"\")"=w464) -> ("States Out"=w463:string)  [unwired: 14 in]
      }
      frame "File: Save ITX" {
        n194 = Unbundle By Name(w493) -> ("file.path"=w486:path, "file.Experiment Folder"=w492:string, "file.device"=w490:string, "file.Comments"=w489:string, "data.Data"=w488:cluster{"Y  Array":dbl[]}[], "data.wavenames"=w487:string[])
        n195 = Build Path(base path=w486, name or relative path=w492) -> (appended path=w491:path)
        n196 = call <userlib>:"LV to ITX XY2 AutoPlot.vi"("filename"=w490, "path"=w491, "Notes"=w489, "Data"=w488, "wavenames (.Vx, etc)"=w487) -> ()  [unwired: 10 in, 1 out]
        n197 = call <vilib>:"Add State(s) to Queue__jki_lib_state_machine.vi"("State(s) in (\"\")"=w496) -> ("States Out"=w495:string)  [unwired: 14 in]
      }
    }
  }
  "error out" <- w1
